vi "filterSignals.vi"(8 "ErrorIn":errorcluster, 9 "FilterSignalsAction":T5, 10 "AnalysisSettings":T1={"Fault Thresholds"={"Parameters labels"=[], "Parameters thresholds"=[], "Freqs and thresholds"=[], "Orders and thresholds"=[]}, "Analysis series name"="Analiza", "Save data analysis?"=TRUE, "F-Band Size"=20, "OrderAnalysis?"=TRUE, "Accelerometer"=enum."MMA7351", "fs [Hz]"=4000.0, "Pulse per revolution"=1, "FFT-Parameters"={"averaging mode"=enum."No averaging", "weighting mode"=enum."Linear", "number of averages"=0}, "O-WindowPowerSpectrum"=0, "O-SpectrumAveraging"=enum."No averaging", "O-MaxOrder"=0.0, "O-Resolution"=0.0, "O-BandSize"=0.0, "FrameLength [s]"=1.0, "Aq.FrameLength [ms]"=0, "FilterOrder"=0, "Sensitivity [V/g]"=[]}, 11 "AccelerationData":waveform(dbl)[](array[waveform])) -> (0 "ErrorOut":errorcluster, 3 "RMS values":dbl[][](array[numeric]))   [LabVIEW 2019]
uses:
  FilterSignalsAction.ctl
  VibrationDiagnosisDesktopApp/mainVIs/DialogsVIs/AnalysisSettings.ctl
  Thresholds.ctl
  FaultParameter.ctl
  aquireAccelerationDataVIs/Accelerometer.ctl
  <vilib>/addons/Digital Filter Design/Process.llb/DFD Filtering (Wfm NChan).vi
  <vilib>/measure/madcrms.llb/Basic Averaged DC-RMS for N Chan.vi
  <vilib>/addons/Digital Filter Design/NI_DigFilterLicensed.lvlib
  <vilib>/measure/NI_MAPro.lvlib
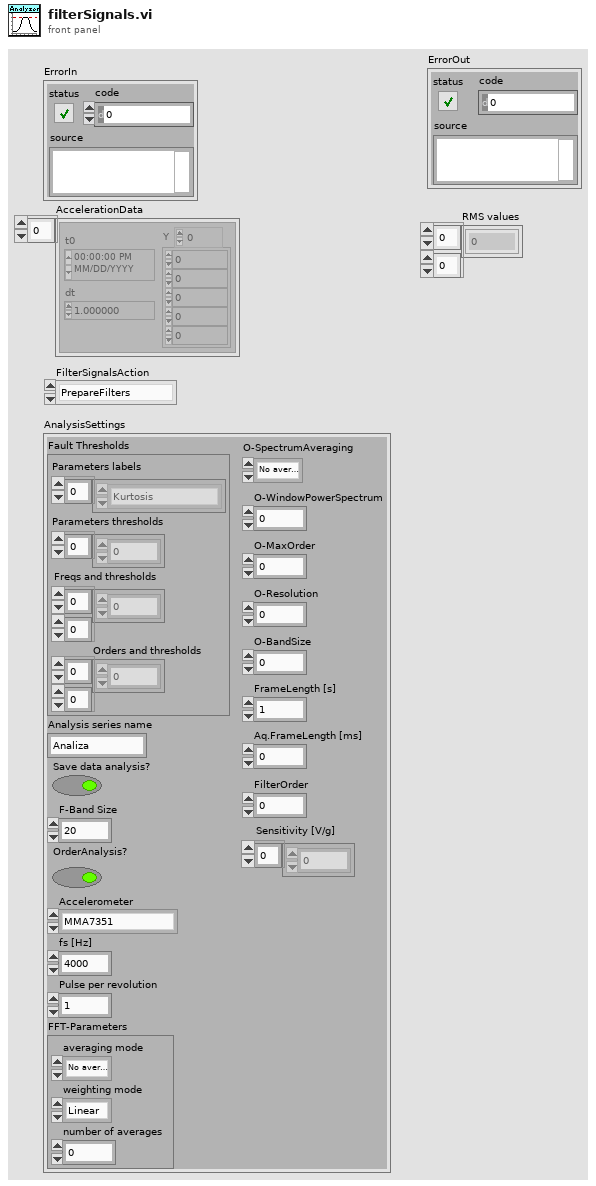
[diagram p1: front panel]
types:
  T1 = typedef "AnalysisSettings.ctl" = cluster{"Fault Thresholds":T2, "Analysis series name":string, "Save data analysis?":bool, "F-Band Size":i32, "OrderAnalysis?":bool, "Accelerometer":T4, "fs [Hz]":dbl, "Pulse per revolution":u16, "FFT-Parameters":cluster{"averaging mode":enum16{"No averaging", "Vector averaging", "RMS averaging", "Peak hold"}, "weighting mode":enum16{"Linear", "Exponential"}, "number of averages":u32}, "O-WindowPowerSpectrum":u32, "O-SpectrumAveraging":enum16{"No averaging", "Vector averaging", "RMS averaging", "Peak hold"}, "O-MaxOrder":dbl, "O-Resolution":dbl, "O-BandSize":dbl, "FrameLength [s]":dbl, "Aq.FrameLength [ms]":i64, "FilterOrder":i32, "Sensitivity [V/g]":dbl[]}
  T2 = typedef "Thresholds.ctl" = cluster{"Parameters labels":T3[], "Parameters thresholds":dbl[], "Freqs and thresholds":dbl[][], "Orders and thresholds":dbl[][]}
  T3 = typedef "FaultParameter.ctl" = enum16{"Kurtosis", "RMS", "Crest factor"}
  T4 = typedef "Accelerometer.ctl" = enum16{"None", "MPU6050", "MMA7351"}
  T5 = typedef "FilterSignalsAction.ctl" = enum16{"PrepareFilters", "Filter"}
  T6 = enum16{"Lowpass", "Highpass", "Bandpass", "Bandstop"}
  T7 = typedef "NI_DigFilterLicensed.lvlib/DFD Filter Obj.ctl" = cluster{"mSRate_Fs":dbl, "mSRate_Version":string, "mSRate_Comments":string, "mSRate_OrgCoef":T8, "mSRate_CurCoef":T8, "mSRate_Quantized?":bool, "mSRate_QCoef":T8, "mSRate_QSettings":T10[], "mSRate_Order":i32, "mSRate_Scaling":cluster{"mSRate_ScaleByPowerOf2?":bool, "mSRate_ScaleType":T12}}
  T8 = typedef "NI_DigFilterLicensed.lvlib/DFD Filter Coef.ctl" = cluster{"type":T9, "gain":dbl, "coef a (k)":dbl[], "coef b (v)":dbl[]}
  T9 = typedef "NI_DigFilterLicensed.lvlib/DFD Filter Structure Type Selector.ctl" = enum16{"Undefined", "FIR Direct Form", "FIR Direct Form Transposed", "FIR Symmetric", "FIR Antisymmetric", "IIR Direct Form I", "IIR Direct Form I Transposed", "IIR Direct Form II", "IIR Direct Form II Transposed", "IIR Cascaded Second Order Sections Form I", "IIR Cascaded Second Order Sections Form I Transposed", "IIR Cascaded Second Order Sections Form II", "IIR Cascaded Second Order Sections Form II Transposed", "Lattice Allpass (basic sections)", "Lattice Allpass (one multiplier sections)", "Lattice Allpass (normalized sections)", "Lattice AR (basic sections)", "Lattice AR (one multiplier sections)", "Lattice AR (normalized sections)", "Lattice MA (minimum phase)", "Lattice MA (maximum phase)", "Lattice ARMA (basic sections)", "Lattice ARMA (one multiplier sections)", "Lattice ARMA (normalized sections)"}
  T10 = typedef "NI_DigFilterLicensed.lvlib/dfd_Internal Quantization Settings.ctl" = cluster{"source":T11, "wl":i16, "iwl":i16, "overflow mode":enum16{"Saturation", "Wrap"}, "rounding mode":enum16{"Nearest", "Truncation"}, "signed?":bool}
  T11 = typedef "NI_DigFilterLicensed.lvlib/dfd_Internal Quantization Srcs.ctl" = u16
  T12 = typedef "NI_DigFilterLicensed.lvlib/DFD Coef Norm Type.ctl" = enum16{"No Norm", "Time Domain 1-Norm", "Time Domain 2-Norm", "Time Domain Inf-Norm"}
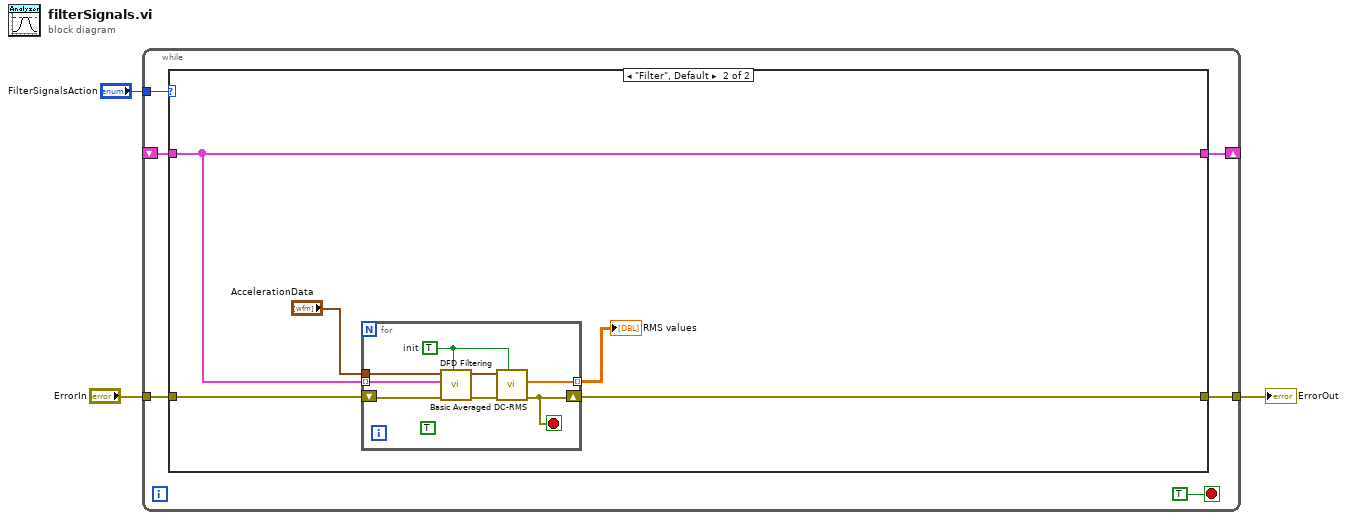
[diagram p0: block diagram]
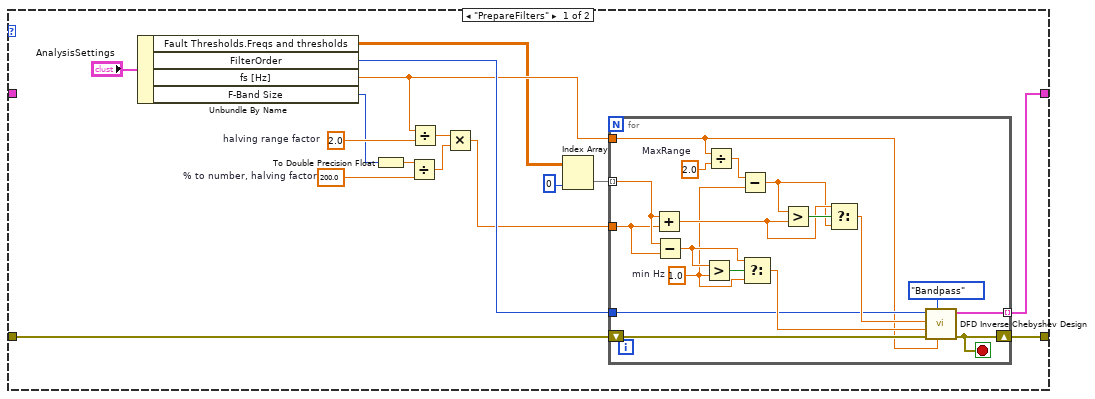
[diagram p2: hidden frame]
diagram:
  n1 = while {
    tunnel: "FilterSignalsAction" -> [w8]
    tunnel: "ErrorIn" -> [w7]
    shift-right: [w6] -> _
    shift-left: _ -> [w4]
    tunnel: [w5] -> w1
    stop <- TRUE stop-if-true
    n2 = case shown="\"Filter\", Default" w8 {
      tunnel: w7 -> [w19 w48]
      tunnel: [w12 w44] -> w6
      tunnel: [w11 w45] -> w5
      tunnel: w4 -> [_ w44]
      frame "PrepareFilters" {
        w23 = 2.0  # halving range factor
        w24 = 200.0  # % to number, halving factor
        n3 = Unbundle By Name("AnalysisSettings") -> ("Fault Thresholds.Freqs and thresholds"=w15:dbl[][], "FilterOrder"=w18:i32, "fs [Hz]"=w17:dbl, "F-Band Size"=w20:i32)
        n4 = To Double Precision Float(number=w20) -> (double precision float=w25:dbl)
        n5 = Divide(x=w25, y=w24) -> (x/y=w21:dbl)
        n6 = Divide(x=w17, y=w23) -> (x/y=w22:dbl)
        n7 = Multiply(x=w22, y=w21) -> (x*y=w13:dbl)
        n8 = Index Array(array=w15, index (col)=0 ("disabled index (col)")) -> (element=w14:dbl[])  [unwired: 1 in]
        n9 = for {
          tunnel: w18 -> [w31]
          tunnel: w17 -> [w28]
          tunnel: w14 -> [w30] mode=indexing
          tunnel: w13 -> [w29]
          tunnel: [w27] -> w12 mode=indexing
          shift-right: [w26] -> w11
          shift-left: w19 -> [w32]
          stop <- w26 stop-if-true
          w33 = 1.0  # min Hz
          w42 = 2.0  # MaxRange
          n10 = Add(x=w30, y=w29) -> (x+y=w36:dbl)
          n11 = Subtract(x=w30, y=w29) -> (x-y=w38:dbl)
          n12 = Greater?(x=w38, y=w33) -> (0:w39:bool)
          n13 = Divide(x=w28, y=w42) -> (x/y=w35:dbl)
          n14 = Subtract(x=w35, y=w33) -> (x-y=w34:dbl)
          n15 = Select(t=w38, s=w39, f=w33) -> (s? t:f=w37:dbl)
          n16 = Greater?(x=w34, y=w36) -> (0:w41:bool)
          n17 = Select(t=w36, s=w41, f=w34) -> (s? t:f=w40:dbl)
          n18 = call <vilib>:"DFD Inverse Chebyshev Design.vi"("fs [Hz]"=w28, "filter type"=T6."Bandpass", "error in (no error)"=w32, "low cutoff freq [Hz]"=w37, "high cutoff freq [Hz]"=w40, "order"=w31) -> ("error out"=w26:errorcluster, "filter out"=w27:T7)  [unwired: 4 in]
        }
      }
      frame "Filter", Default {
        n19 = for {
          tunnel: "AccelerationData" -> [w53]
          tunnel: w44 -> [w52] mode=indexing
          tunnel: [w50] -> w46 mode=indexing
          shift-right: [w49] -> w45
          shift-left: w48 -> [w51]
          stop <- w49 stop-if-true
          w54 = TRUE  # init
          (unwired) TRUE ("init/cont (init:F)")
          n20 = call-poly <vilib>:"DFD Filtering.vi"("init? (F)"=w54, "error in (no error)"=w51, "filter"=w52, "signal in"=w53) -> ("error out"=w55:errorcluster, "signal out"=w56:waveform(dbl)[])  [unwired: 6 in]
          n21 = call-poly <vilib>:"Basic Averaged DC-RMS.vi"("reset"=w54, "error in (no error)"=w55, "signals in"=w56) -> ("error out"=w49:errorcluster, "RMS values"=w50:dbl[])  [unwired: 5 in, 2 out]
        }
        "RMS values" <- w46
      }
    }
  }
  "ErrorOut" <- w1
